vi "User.SettingsGui.vi"(11 "User in":i32(ring) caption="Operator" items=["-", "Admin", "Maciek"]) -> ()   [LabVIEW 2013]
uses:
  User.Global.vi
  User.SettingsGui.Action.ctl
  User.Level.ctl
  Tma.lib/array.llb/Select I32s from array.vi
  Tma.lib/array.llb/Select strings from array.vi
  EventLog/EventLog.New(array).vi
  Translator/Translator.Message.ctl
panel:
  out "_loop":i32(ring)=4
  in  "open?":bool
  in  "NewButton":bool
  in  "GuruPeriod":u32 caption="Guru Period Time [day]"
  in  "SetGuru":bool caption="Guru"
  in  "CancelButton":bool
  in  "UserLevel":T1 caption="User Level"
  in  "AutoLogOffTime":u32=1 caption="Auto Log-Off Time [min]" min=1 max=9999
  in  "RemoveButton":bool
  in  "ModifyButton":bool
  in  "AddButton":bool
  in  "UserName":string caption="Name"
  in  "pwd_Password2":string caption="Confirm Password"
  in  "pwd_Password":string caption="Password"
  in  "User":i32(ring) caption="Operator" items=["Service"=1, "Operator"=2]
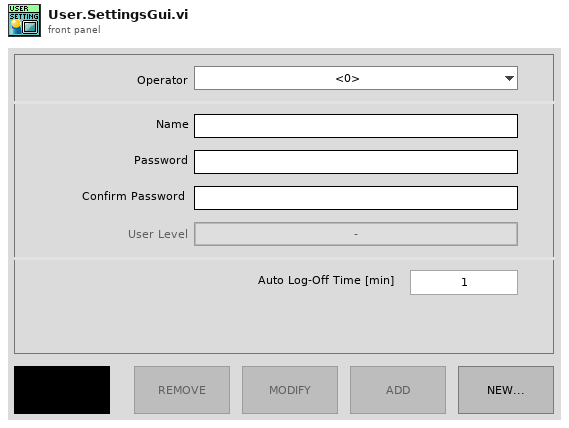
[diagram p1: front panel]
types:
  T1 = typedef "User.Level.ctl" = enum16{"-", "Operator", "Technician", "Administrator"}
  T2 = typedef "User.SettingsGui.Action.ctl" = enum32{"idle", "constructor", "destructor", "--- User Settings GUI ---", "check name & pass", "add user", "modify user", "remove user", "select user"}
  T3 = typedef "Translator.Message.ctl" = enum16{"-", "Event confirmed", "Log out", "Log in", "Shutdown", "Cancel", "Start", "Error %d >> %s", "Error %d >> %s >> %s", "Starting %s", "Quitting %s", "User %s level %s added", "User %s level %s deleted", "User %s level %s changed to %s", "Configured", "Initializing", "Quitting", "Loading", "Running", "Stopped", "Do you want to continue?", "Calibration", "Log out?", "System", "All", "IDLE", "Translating...%s", "Not found", "Alarm %s", "Restart is required to translate the application! Do you want to restart the PC?", "Restart cancelled. Be aware that some controls may not be fully translated until you restart the application.", "New version available!", "The software is up-to-date", "PC software will be updated after rebooting the PC. Do you want to reboot now?", "RT software will be updated. Make sure that no process is running. Do you want to reboot RT now?", "Updating RT firmware. Please wait...", "Update failed: %s", "Rebooting...", "Rebooting RT. Please wait...", "RT updated to version %s", "Timeout error during update. Check if RT is working", "Run", "Skip", "Abort", "Please wait...", "Database disconnected - changeover disabled!", "Put reference number...", "Folder '%s' is missing", "File '%s' is missing", "File '%s' is broken", "File '%s' is running", "Log file '%s' started", "Step '%s' added to log file", "Log file '%s' ended", "Test steps are missing", "Output %s = %.3f", "Process param '%s' not found in DB", "Process param '%s' wrong order", "Process param '%s' value %.3f out of limits (%.3f; %.3f)", "Step%d param '%s' not found in DB", "Step%d param '%s' wrong order", "Step%d param '%s' value %.3f out of limits (%.3f; %.3f)", "Step%d EV '%s' not found in DB", "Step%d EV '%s' wrong order", "Reference %d accepted", "Scan label failed", "Scan label failed. Error %d", "Scan label failed. Scanner disconnected", "Scan label: %s, %s", "Scan plate failed", "Scan plate failed. Wrong reference %d", "Scan plate failed. Serial number %d not unique", "Scan plate failed. Error %s", "Scan plate failed. Scanner disconnected", "Scan plate: %d", "DAQ.DO '%s' = %d", "DAQ.DI '%s' = %d->%d", "CPX.DO '%s' = %d", "CPX.DOvalve '%s' = %d", "CPX.DI '%s' = %d->%d", "Unable to move Door to %s position - timeout", "Unable to move Door to %s position - emergency button", "Unable to move Door to %s position - safety bar", "Unable to move Door to %s position - safety edge", "Unable to reset Emergency Circuit - emg button", "Unable to reset Emergency Circuit - safety bar", "Unable to set digital output '%s' = %d", "Unable to switch on Air Main Valve - timeout", "Unable to switch off Air Main Valve - timeout", "Unable to move Servo Lift to %s position - timeout", "Unable to move Servo Lift to %s position - air pressure off", "Unable to move Product Press to %s position - timeout", "Unable to move Product Press to %s position - air pressure off", "Unable to move Needles to %s position - timeout", "Unable to move Needles to %s position - air pressure off", "Unable to move Plugs to %s position - timeout", "Unable to move Plugs to %s position - air pressure off", "Unable to move Plugs to %s position - Plug Press not in Home position", "Unable to move Screw to %s position - timeout", "Unable to move Screw to %s position - air pressure off", "Unable to move Plug Revolver to %s position - timeout", "Unable to move Plug Revolver to %s position - air pressure off", "Unable to move Plug Revolver to %s position - Plug Press not in Home position", "Unable to reload Plug Revolver - magazine missing", "Unable to reload Plug Revolver - magazine empty", "Reloaded last plugs in Plug Revolver", "Unable to move Plug Press to %s position while getting plugs from revolver - timeout", "Unable to move Plug Press to %s position while pressing plugs into product - timeout", "Unable to move Plug Press to %s position - undefined position of Plugs", "Unable to move Plug Press to %s position - air pressure off", "Unable to move Stamp to %s position - timeout", "Unable to move Stamp to %s position - air pressure off", "Unable to move Vent Press to %s position - timeout", "Unable to move Vent Press to %s position - air pressure off", "Unable to move Terminal Press to %s position - timeout", "Unable to move Terminal Press to %s position - air pressure off"}
  T4 = enum32{"invalid app kind", "Development System", "Run Time System", "Student Edition", "Embedded LabVIEW", "Evaluation", "Custom"}
  T5 = enum8{"Enabled", "Disabled", "Disabled and Grayed Out"}
  T6 = typedef "User.Info.ctl" = cluster{"ID":i32, "Name":string, "Pass":string, "Level":T1, "Del":bool}
  T7 = typedef "LVStringsAndValuesArrayTypeDef_I32.ctl" = cluster{"String":string, "Value":i32}[]
  T8 = typedef "LVPositionTypeDef.ctl" = cluster{"Left":i32, "Top":i32}
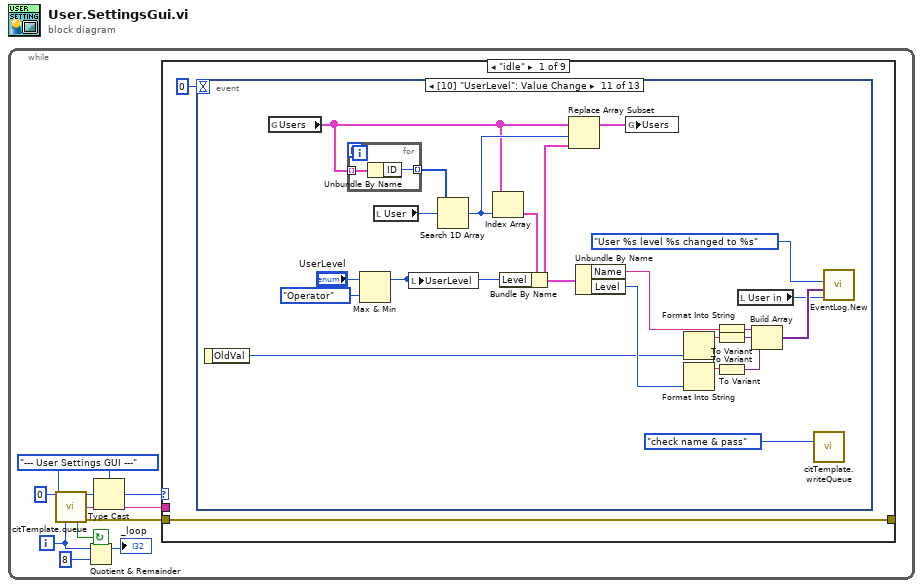
[diagram p0: block diagram]
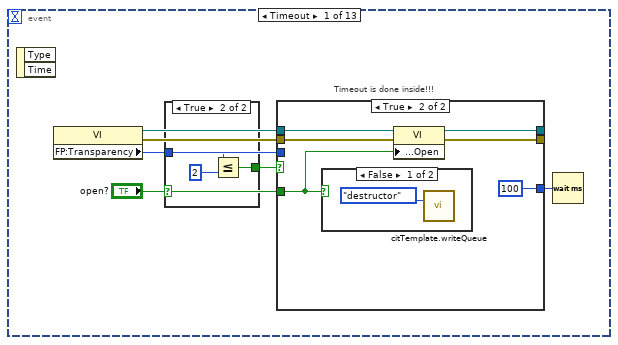
[diagram p2: hidden frame]
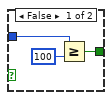
[diagram p3: hidden frame]
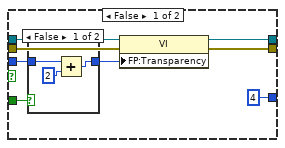
[diagram p4: hidden frame]
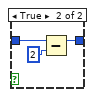
[diagram p5: hidden frame]
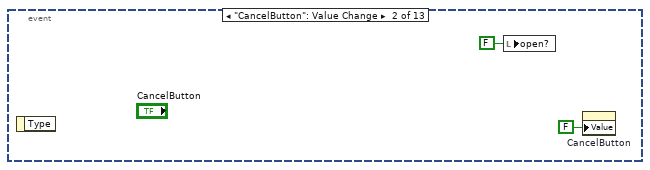
[diagram p7: hidden frame]
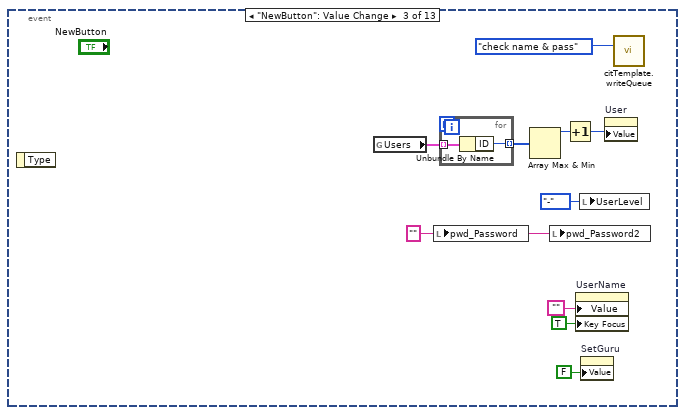
[diagram p8: hidden frame]
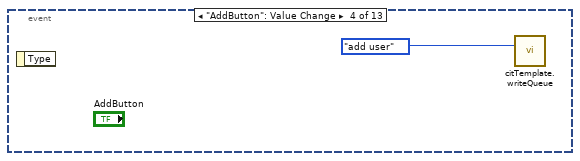
[diagram p9: hidden frame]
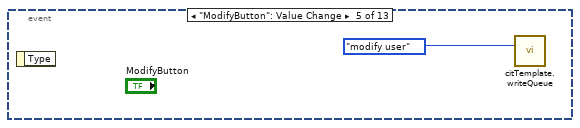
[diagram p10: hidden frame]
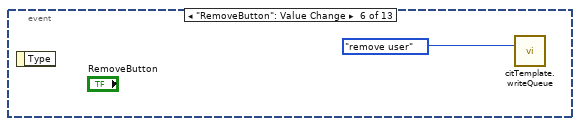
[diagram p11: hidden frame]
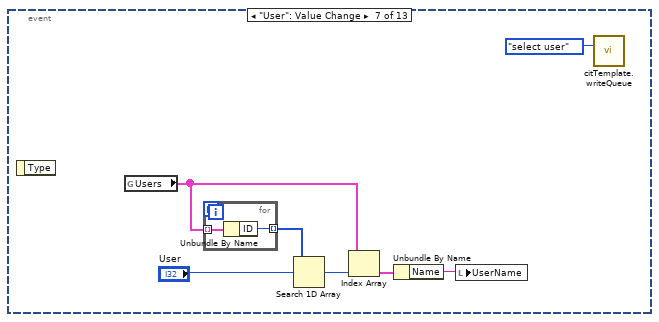
[diagram p12: hidden frame]
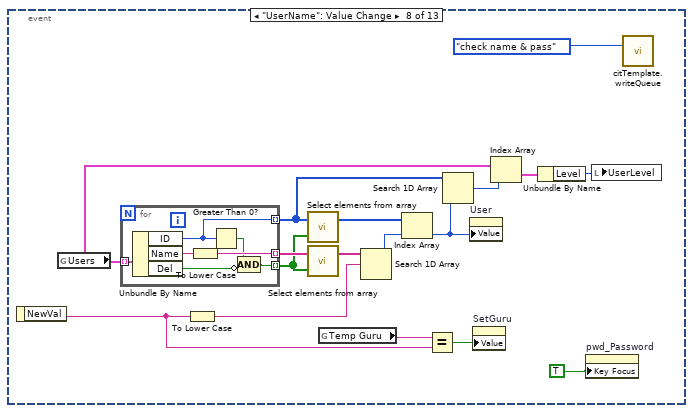
[diagram p13: hidden frame]
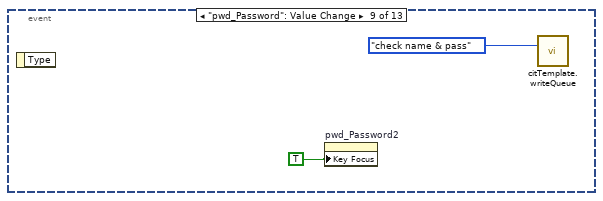
[diagram p14: hidden frame]
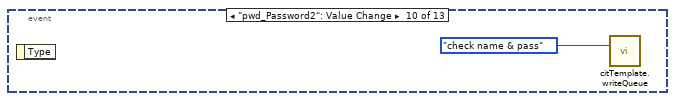
[diagram p15: hidden frame]
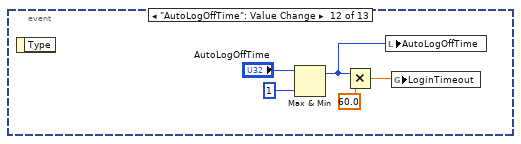
[diagram p16: hidden frame]
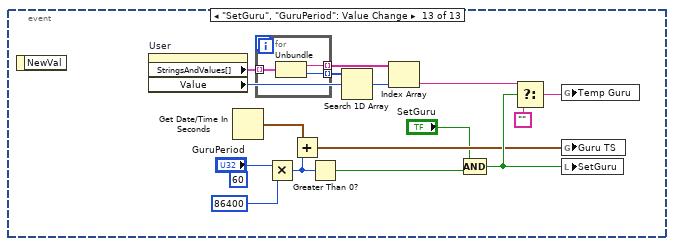
[diagram p17: hidden frame]
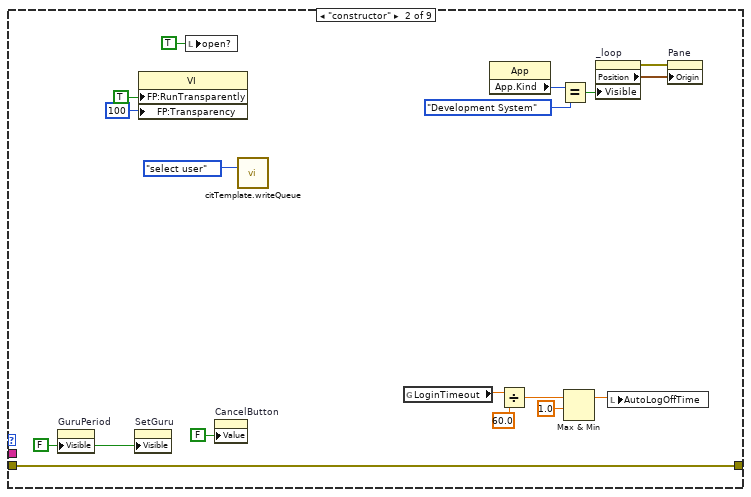
[diagram p18: hidden frame]
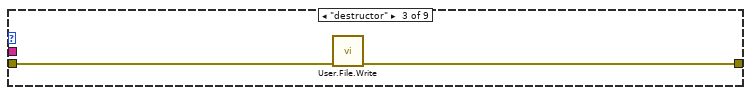
[diagram p19: hidden frame]
diagram:
  n1 = while {
    i -> [w1]
    stop <- w7 continue-if-true
    w6 = User.SettingsGui.Action."--- User Settings GUI ---" ("Action")
    n2 = call "citTemplate.queue.vi"("ms timeout (250 ms)"=0, "event enum"=w6, "iteration (-1)"=w1) -> ("event out"=w10:u32, "(flatten) data out"=w9:string, "continue"=w7:bool, "error out"=w8:errorcluster)  [unwired: 2 in, 7 out]
    n3 = Quotient & Remainder(x=w1, y=8) -> (x-y*floor(x/y)=→"_loop":i32)  [unwired: 1 out]
    n4 = Type Cast(type=w6, x=w10) -> (*(type *) &x=w5:T2)
    n5 = case shown="\"idle\"" w5 {
      tunnel: w9 -> [_ _ _ _ _ _ _ _ _]
      tunnel: w8 -> [w11 w147 w164 w166 w204 w259 w305 w332 w366]
      tunnel: [w11 w147 w165 w166 w204 w259 w305 w332 w366] -> _
      frame "idle" {
        n6 = event shown="[10] \"UserLevel\": Value Change" {
          selector: _ -> [_ _ _ _ _ _ _ _ _ _ _ _ _]
          dyn-events: _ -> [_ _ _ _ _ _ _ _ _ _ _ _ _]
          timeout: 0 -> [_ _ _ _ _ _ _ _ _ _ _ _ _]
          event Timeout {
            # "Timeout is done inside!!!"
            n7 = event-data() -> ()  [unwired: 1 in, 2 out]
            n8 = property class="VI"() -> (reference out=w16:refnum<vi>, error out=w15:errorcluster, "FP:Transparency"=w17:u8)  [unwired: 2 in]
            n9 = case shown="True" "open?" {
              tunnel: w17 -> [w20 w24]
              tunnel: [w19 w23] -> w18
              frame False {
                n10 = Greater Or Equal?(x=w20, y=u8 100) -> (x >= y?=w19:bool)
              }
              frame True {
                n11 = Less Or Equal?(x=w24, y=u8 2) -> (x <= y?=w23:bool)
              }
            }
            n12 = case shown="True" w18 {
              tunnel: w15 -> [w32 w44]
              tunnel: w16 -> [w31 w43]
              tunnel: w17 -> [w30 _]
              tunnel: "open?" -> [w29 w39]
              tunnel: [w27 w42] -> _
              tunnel: [w26 w41] -> _
              tunnel: [u32 4 ("milliseconds to wait") u32 100 ("ms timeout (250 ms)")] -> w13
              frame False {
                n13 = case shown="False" w29 {
                  tunnel: w30 -> [w35 w37]
                  tunnel: [w34 w36] -> w28
                  frame False {
                    n14 = Add(x=w35, y=u8 2 ("x")) -> (x+y=w34:u8)
                  }
                  frame True {
                    n15 = Subtract(x=w37, y=u8 2 ("x")) -> (x-y=w36:u8)
                  }
                }
                n16 = property class="VI"(reference=w31, error in=w32, "FP:Transparency"=w28) -> (reference out=w26:refnum<vi>, error out=w27:errorcluster)
              }
              frame True {
                n17 = case shown="False" w39 {
                  frame False {
                    n18 = call "citTemplate.writeQueue.vi"("event in (if not connected:all statemachine with data event)"=User.SettingsGui.Action."destructor" ("Action")) -> ()  [unwired: 4 in, 11 out]
                  }
                  frame True {
                  }
                }
                n19 = property class="VI"(reference=w43, error in=w44, "Front Panel.Open"=w39) -> (reference out=w41:refnum<vi>, error out=w42:errorcluster)
              }
            }
            n20 = Wait (ms)(milliseconds to wait=w13) -> ()  [unwired: 1 out]
          }
          event "CancelButton": Value Change {
            n21 = event-data() -> ()  [unwired: 1 in, 1 out]
            n22 = local write "open?"(FALSE ("open?")) -> ()
            n23 = property on="CancelButton" class="Bool (strict)"("Value"=FALSE ("CancelButton")) -> ()  [unwired: 2 in, 2 out]
          }
          event "NewButton": Value Change {
            w56 = "" ("Password")
            n24 = event-data() -> ()  [unwired: 1 in, 1 out]
            n25 = global read "User.Global.vi" "Users"() -> (w51:T6[])
            n26 = local write "pwd_Password"(w56) -> ()
            n27 = for {
              tunnel: w51 -> [w59] mode=indexing
              tunnel: [w58] -> w50 mode=indexing
              n28 = Unbundle By Name(w59) -> ("ID"=w58:i32)
            }
            n29 = Array Max & Min(array=w50) -> (max value=w49:i32)  [unwired: 3 out]
            n30 = local write "pwd_Password2"(w56) -> ()
            n31 = Increment(x=w49) -> (x+1=w48:i32)
            n32 = property on="UserName" class="Str"("Value"="", "Key Focus"=TRUE) -> ()  [unwired: 2 in, 2 out]
            n33 = local write "UserLevel"(User.Level."-" ("UserLevel")) -> ()
            n34 = property on="SetGuru" class="Bool (strict)"("Value"=FALSE ("SetGuru")) -> ()  [unwired: 2 in, 2 out]
            n35 = property on="User" class="Ring (strict)"("Value"=w48) -> ()  [unwired: 2 in, 2 out]
            n36 = call "citTemplate.writeQueue.vi"("event in (if not connected:all statemachine with data event)"=User.SettingsGui.Action."check name & pass" ("Action")) -> ()  [unwired: 14 in, 1 out]
          }
          event "AddButton": Value Change {
            n37 = event-data() -> ()  [unwired: 1 in, 1 out]
            n38 = call "citTemplate.writeQueue.vi"("event in (if not connected:all statemachine with data event)"=User.SettingsGui.Action."add user" ("Action")) -> ()  [unwired: 14 in, 1 out]
          }
          event "ModifyButton": Value Change {
            n39 = event-data() -> ()  [unwired: 1 in, 1 out]
            n40 = call "citTemplate.writeQueue.vi"("event in (if not connected:all statemachine with data event)"=User.SettingsGui.Action."modify user" ("Action")) -> ()  [unwired: 14 in, 1 out]
          }
          event "RemoveButton": Value Change {
            n41 = event-data() -> ()  [unwired: 1 in, 1 out]
            n42 = call "citTemplate.writeQueue.vi"("event in (if not connected:all statemachine with data event)"=User.SettingsGui.Action."remove user" ("Action")) -> ()  [unwired: 14 in, 1 out]
          }
          event "User": Value Change {
            n43 = event-data() -> ()  [unwired: 1 in, 1 out]
            n44 = global read "User.Global.vi" "Users"() -> (w65:T6[])
            n45 = for {
              tunnel: w65 -> [w71] mode=indexing
              tunnel: [w70] -> w67 mode=indexing
              n46 = Unbundle By Name(w71) -> ("ID"=w70:i32)
            }
            n47 = Search 1D Array(1D array=w67, element="User") -> (index of element=w66:i32)  [unwired: 1 in]
            n48 = Index Array(array=w65, index=w66) -> (element=w64:T6)
            n49 = Unbundle By Name(w64) -> ("Name"=w68:string)
            n50 = local write "UserName"(w68) -> ()
            n51 = call "citTemplate.writeQueue.vi"("event in (if not connected:all statemachine with data event)"=User.SettingsGui.Action."select user" ("Action")) -> ()  [unwired: 14 in, 1 out]
          }
          event "UserName": Value Change {
            n52 = event-data() -> ("NewVal"=w77:string)  [unwired: 1 in]
            n53 = global read "User.Global.vi" "Users"() -> (w73:T6[])
            n54 = for {
              tunnel: w73 -> [w95] mode=indexing
              tunnel: [w93] -> w84 mode=indexing
              tunnel: [w91] -> w72 mode=indexing
              tunnel: [w89] -> w75 mode=indexing
              n55 = Unbundle By Name(w95) -> ("ID"=w89:i32, "Name"=w94:string, "Del"=w92:bool)
              n56 = To Lower Case(string=w94) -> (all lower case string=w93:string)
              n57 = Greater Than 0?(x=w89) -> (x > 0?=w90:bool)
              n58 = Compound Arithmetic op=AND(w90, invert w92) -> (w91:bool)
            }
            n59 = To Lower Case(string=w77) -> (all lower case string=w87:string)
            n60 = call-poly "Select elements from array.vi"("selection array"=w72, "I32s"=w75) -> ("selected I32s"=w82:i32[])  [unwired: 1 in]
            n61 = call-poly "Select elements from array.vi"("selection array"=w72, "strings"=w84) -> ("selected strings"=w83:string[])  [unwired: 1 in]
            n62 = global read "User.Global.vi" "Temp Guru"() -> (w80:string)
            n63 = Search 1D Array(1D array=w83, element=w87) -> (index of element=w81:i32)  [unwired: 1 in]
            n64 = Index Array(array=w82, index=w81) -> (element=w76:i32)
            n65 = Equal?(x=w80, y=w77) -> (x = y?=w79:bool)
            n66 = Search 1D Array(1D array=w75, element=w76) -> (index of element=w74:i32)  [unwired: 1 in]
            n67 = property on="User" class="Ring (strict)"("Value"=w76) -> ()  [unwired: 2 in, 2 out]
            n68 = property on="SetGuru" class="Bool (strict)"("Value"=w79) -> ()  [unwired: 2 in, 2 out]
            n69 = Index Array(array=w73, index=w74) -> (element=w86:T6)
            n70 = Unbundle By Name(w86) -> ("Level"=w85:T1)
            n71 = property on="pwd_Password" class="Str"("Key Focus"=TRUE) -> ()  [unwired: 2 in, 2 out]
            n72 = local write "UserLevel"(w85) -> ()
            n73 = call "citTemplate.writeQueue.vi"("event in (if not connected:all statemachine with data event)"=User.SettingsGui.Action."check name & pass" ("Action")) -> ()  [unwired: 14 in, 1 out]
          }
          event "pwd_Password": Value Change {
            n74 = event-data() -> ()  [unwired: 1 in, 1 out]
            n75 = property on="pwd_Password2" class="Str"("Key Focus"=TRUE) -> ()  [unwired: 2 in, 2 out]
            n76 = call "citTemplate.writeQueue.vi"("event in (if not connected:all statemachine with data event)"=User.SettingsGui.Action."check name & pass" ("Action")) -> ()  [unwired: 14 in, 1 out]
          }
          event "pwd_Password2": Value Change {
            n77 = event-data() -> ()  [unwired: 1 in, 1 out]
            n78 = call "citTemplate.writeQueue.vi"("event in (if not connected:all statemachine with data event)"=User.SettingsGui.Action."check name & pass" ("Action")) -> ()  [unwired: 14 in, 1 out]
          }
          event Value Change {
            n79 = event-data() -> ("OldVal"=w101:T1)  [unwired: 1 in]
            n80 = global read "User.Global.vi" "Users"() -> (w112:T6[])
            n81 = for {
              tunnel: w112 -> [w122] mode=indexing
              tunnel: [w121] -> w115 mode=indexing
              n82 = Unbundle By Name(w122) -> ("ID"=w121:i32)
            }
            n83 = Max & Min(x="UserLevel", y=User.Level."Operator") -> (max(x,y)=w118:u16)  [unwired: 1 out]
            n84 = local read "User"() -> (w114:i32)
            n85 = local write "UserLevel"(w118) -> ()
            n86 = Search 1D Array(1D array=w115, element=w114) -> (index of element=w113:i32)  [unwired: 1 in]
            n87 = Index Array(array=w112, index=w113) -> (element=w104:T6)
            n88 = Bundle By Name(cluster=w104, "Level"=w118) -> (w103:T6)
            n89 = Replace Array Subset(array=w112, new element=w103, index=w113) -> (w116:T6[])
            n90 = Unbundle By Name(w103) -> ("Name"=w105:string, "Level"=w102:T1)
            n91 = global write "User.Global.vi" "Users"(w116) -> ()
            n92 = Format Into String(w101) -> (resulting string=w110:string)  [unwired: 3 in, 1 out]
            n93 = Format Into String(w102) -> (resulting string=w100:string)  [unwired: 3 in, 1 out]
            n94 = To Variant(anything=w105) -> (Variant=w109:variant)
            n95 = To Variant(anything=w110) -> (Variant=w108:variant)
            n96 = To Variant(anything=w100) -> (Variant=w99:variant)
            n97 = local read "User in"() -> (w106:i32)
            n98 = Build Array(w109, w108, w99) -> (w107:variant[])
            n99 = call "citTemplate.writeQueue.vi"("event in (if not connected:all statemachine with data event)"=User.SettingsGui.Action."check name & pass" ("Action")) -> ()  [unwired: 14 in, 1 out]
            n100 = call-poly "EventLog.New.vi"("error in (no error)"=w106, "Arguments"=w107, "Message (-)"=Translator.Message."User %s level %s changed to %s") -> ()  [unwired: 7 in, 2 out]
          }
          event "AutoLogOffTime": Value Change {
            n101 = event-data() -> ()  [unwired: 1 in, 1 out]
            n102 = Max & Min(x="AutoLogOffTime", y=u32 1 ("lower limit")) -> (max(x,y)=w127:u32)  [unwired: 1 out]
            n103 = Multiply(x=w127, y=60.0 ("x")) -> (x*y=w123:dbl)
            n104 = local write "AutoLogOffTime"(w127) -> ()
            n105 = global write "User.Global.vi" "LoginTimeout"(w123) -> ()
          }
          event "SetGuru", "GuruPeriod": Value Change {
            (unwired) u32 60 ("y")
            n106 = event-data() -> ()  [unwired: 1 in, 1 out]
            n107 = property on="User" class="Ring (strict)"() -> ("StringsAndValues[]"=w133:T7, "Value"=w131:i32)  [unwired: 2 in, 2 out]
            n108 = Get Date/Time In Seconds() -> (seconds since 1Jan1904=w134:timestamp)
            n109 = for {
              tunnel: w133 -> [w146] mode=indexing
              tunnel: [w145] -> w132 mode=indexing
              tunnel: [w144] -> w130 mode=indexing
              n110 = Unbundle(w146) -> ("String"=w144:string, "Value"=w145:i32)
            }
            n111 = Multiply(x="GuruPeriod", y=u32 86400) -> (x*y=w135:u32)
            n112 = Add(x=w134, y=w135) -> (x+y=w140:timestamp)
            n113 = Greater Than 0?(x=w135) -> (x > 0?=w137:bool)
            n114 = Search 1D Array(1D array=w132, element=w131) -> (index of element=w129:i32)  [unwired: 1 in]
            n115 = Index Array(array=w130, index=w129) -> (element=w128:string)
            n116 = Compound Arithmetic op=AND("SetGuru", w137) -> (w141:bool)
            n117 = Select(t=w128, s=w141, f="") -> (s? t:f=w136:string)
            n118 = global write "User.Global.vi" "Temp Guru"(w136) -> ()
            n119 = global write "User.Global.vi" "Guru TS"(w140) -> ()
            n120 = local write "SetGuru"(w141) -> ()
          }
        }
      }
      frame "constructor" {
        w157 = FALSE ("Visible")
        n121 = property on="GuruPeriod" class="DigNum (strict)"("Visible"=w157) -> ()  [unwired: 2 in, 2 out]
        n122 = property on="SetGuru" class="Bool (strict)"("Visible"=w157) -> ()  [unwired: 2 in, 2 out]
        n123 = property class="VI"("FP:RunTransparently"=TRUE ("Front Panel Window:Run VI Transparently"), "FP:Transparency"=u8 100 ("Front Panel Window:Transparency")) -> ()  [unwired: 2 in, 2 out]
        n124 = local write "open?"(TRUE ("open?")) -> ()
        n125 = property on="CancelButton" class="Bool (strict)"("Value"=FALSE ("CancelButton")) -> ()  [unwired: 2 in, 2 out]
        n126 = call "citTemplate.writeQueue.vi"("event in (if not connected:all statemachine with data event)"=User.SettingsGui.Action."select user" ("Action")) -> ()  [unwired: 14 in, 1 out]
        n127 = global read "User.Global.vi" "LoginTimeout"() -> (w156:dbl)
        n128 = property class="App"() -> ("App.Kind"=w150:T4)  [unwired: 2 in, 2 out]
        n129 = Divide(x=w156, y=60.0 ("x")) -> (x/y=w160:dbl)
        n130 = Equal?(x=w150, y=T4."Development System") -> (x = y?=w148:bool)
        n131 = Max & Min(x=w160, y=1.0 ("lower limit")) -> (max(x,y)=w163:dbl)  [unwired: 1 out]
        n132 = property on="_loop" class="Ring (strict)"("Visible"=w148) -> (error out=w152:errorcluster, "Position"=w151:T8)  [unwired: 2 in, 1 out]
        n133 = local write "AutoLogOffTime"(w163) -> ()
        n134 = property on="Pane" class="Pane"(error in=w152, "Origin"=w151) -> ()  [unwired: 1 in, 2 out]
      }
      frame "destructor" {
        n135 = call "User.File.Write.vi"("error in (no error)"=w164) -> ("error out"=w165:errorcluster)  [unwired: 10 in]
      }
      frame "--- User Settings GUI ---" {
      }
      frame "check name & pass" {
        w194 = User.Level."Administrator" ("x")
        w225 = T5."Disabled and Grayed Out" ("Disabled")
        n136 = global read "User.Global.vi" "Users"() -> (w218:T6[])
        n137 = global read "User.Global.vi" "DefaultUser"() -> (w175:string)
        n138 = global read "User.Global.vi" "Admin User"() -> (w173:string)
        n139 = local read "UserLevel"() -> (w192:T1)
        n140 = for {
          tunnel: w218 -> [w245] mode=indexing
          tunnel: [w243] -> w174 mode=indexing
          tunnel: [w242] -> w212 mode=indexing
          tunnel: [w238] -> w169 mode=indexing
          tunnel: w194 -> [w240]
          tunnel: [w237] -> w193 mode=indexing
          i -> [w236]
          n141 = Greater Than 0?(x=w236) -> (x > 0?=w235:bool)
          n142 = Unbundle By Name(w245) -> ("Level"=w241:T1, "Del"=w238:bool, "Name"=w244:string, "Pass"=w242:string)
          n143 = Equal?(x=w240, y=w241) -> (x = y?=w239:bool)
          n144 = To Lower Case(string=w244) -> (all lower case string=w243:string)
          n145 = Compound Arithmetic op=AND(w235, w239, invert w238) -> (w237:bool)
        }
        n146 = To Lower Case(string="UserName") -> (all lower case string=w213:string)
        n147 = call "MD5 string.vi"("Message String"="pwd_Password") -> ("MD5 message-digest"=w210:string)  [unwired: 10 in]
        n148 = Not Equal?(x="pwd_Password", y="pwd_Password2") -> (x != y?=w229:bool)
        n149 = Empty String/Path?(string/path="pwd_Password") -> (empty?=w228:bool)
        n150 = Equal To 0?(x="User in") -> (x = 0?=w171:bool)
        n151 = Boolean To (0,1)(Boolean=w193) -> (0, 1=w199:i16[])
        n152 = Search 1D Array(1D array=w212, element=w210) -> (index of element=w209:i32)  [unwired: 1 in]
        n153 = Delete From Array(array=w169, index=0) -> (array with subset deleted=w168:bool[])  [unwired: 1 in, 1 out]
        n154 = To Lower Case(string=w175) -> (all lower case string=w177:string)
        n155 = To Lower Case(string=w173) -> (all lower case string=w176:string)
        n156 = Search 1D Array(1D array=w174, element=w213) -> (index of element=w170:i32)  [unwired: 1 in]
        n157 = Array Size(array=w174) -> (size(s)=w224:i32)
        n158 = To Long Integer(number=w199) -> (32bit integer=w198:i32[])
        n159 = Not Equal?(x=w170, y=w209) -> (x != y?=w208:bool)
        n160 = Index Array(array=w169, index=w170) -> (element=w205:bool)
        n161 = Greater Or Equal To 0?(x=w209) -> (x >= 0?=w207:bool)
        n162 = Equal?(x=w213, y=w177) -> (x = y?=w186:bool)
        n163 = Equal?(x=w213, y=w176) -> (x = y?=w179:bool)
        n164 = Add Array Elements(numeric array=w198) -> (sum=w197:i32)
        n165 = Less Or Equal To 0?(x=w224) -> (x <= 0?=w183:bool)
        n166 = Greater Or Equal To 0?(x=w170) -> (x >= 0?=w215:bool)
        n167 = Less Or Equal To 0?(x=w192) -> (x <= 0?=w203:bool)
        n168 = Compound Arithmetic op=AND(w208, w207) -> (w206:bool)
        n169 = And Array Elements(Boolean array=w168) -> (logical AND=w184:bool)
        n170 = Equal?(x=1, y=w197) -> (x = y?=w195:bool)
        n171 = Equal?(x=w194, y=w192) -> (x = y?=w185:bool)
        n172 = Compound Arithmetic op=AND(invert w205, w215) -> (w178:bool)
        n173 = Compound Arithmetic op=OR(w184, w183) -> (w182:bool)
        n174 = Compound Arithmetic op=AND(w185, w195) -> (w180:bool)
        n175 = Compound Arithmetic op=OR(w182, w186, w179, w228, w229, w206) -> (w227:bool)
        n176 = Compound Arithmetic op=OR(w178, w186, w179, w228, w229, w203) -> (w232:bool)
        n177 = Compound Arithmetic op=OR(w180, w182) -> (w181:bool)
        n178 = Compound Arithmetic op=AND(w178, invert w227, invert w203) -> (w226:bool)
        n179 = property on="SetGuru" class="Bool (strict)"() -> ("Value"=w187:bool)  [unwired: 2 in, 2 out]
        n180 = Compound Arithmetic op=AND(w171, w185, invert w182, w178) -> (w191:bool)
        n181 = Select(t=w225, s=w232, f=T5."Enabled" ("Disabled")) -> (s? t:f=w234:T5)
        n182 = Select(t=T5."Disabled and Grayed Out" ("Disabled"), s=w181, f=T5."Enabled" ("Disabled")) -> (s? t:f=w222:T5)
        n183 = property on="GuruPeriod" class="DigNum (strict)"("Visible"=w191) -> ()  [unwired: 2 in, 2 out]
        n184 = Select(t=T5."Enabled" ("Disabled"), s=w226, f=w225) -> (s? t:f=w231:T5)
        n185 = Select(t=T5."Disabled and Grayed Out" ("Disabled"), s=w182, f=T5."Enabled" ("Disabled")) -> (s? t:f=w221:T5)
        n186 = Compound Arithmetic op=AND(invert w185, w187) -> (w190:bool)
        n187 = Select(t=T5."Disabled and Grayed Out" ("Disabled"), s=w180, f=T5."Enabled" ("Disabled")) -> (s? t:f=w202:T5)
        n188 = property on="User" class="Ring (strict)"("DisabledEnum"=w221) -> ()  [unwired: 2 in, 2 out]
        n189 = property on="ModifyButton" class="Bool"("DisabledEnum"=w231) -> ()  [unwired: 2 in, 2 out]
        n190 = property on="AddButton" class="Bool"("DisabledEnum"=w234) -> ()  [unwired: 2 in, 2 out]
        n191 = property on="RemoveButton" class="Bool"("DisabledEnum"=w222) -> ()  [unwired: 2 in, 2 out]
        n192 = Select(t=FALSE, s=w190, f=w187) -> (s? t:f=w188:bool)
        n193 = property on="UserLevel" class="Enum (strict)"("DisabledEnum"=w202) -> ()  [unwired: 2 in, 2 out]
        n194 = property on="SetGuru" class="Bool (strict)"("Value"=w188, "Visible"=w191) -> ()  [unwired: 2 in, 2 out]
      }
      frame "add user" {
        n195 = global read "User.Global.vi" "Users"() -> (w262:T6[])
        n196 = for {
          tunnel: w262 -> [w288] mode=indexing
          tunnel: [w286] -> w264 mode=indexing
          tunnel: [w285] -> w258 mode=indexing
          n197 = Unbundle By Name(w288) -> ("Name"=w287:string, "ID"=w285:i32)
          n198 = To Lower Case(string=w287) -> (all lower case string=w286:string)
        }
        n199 = local read "pwd_Password"() -> (w266:string)
        n200 = local read "UserName"() -> (w250:string)
        n201 = local read "UserLevel"() -> (w252:T1)
        n202 = Array Max & Min(array=w258) -> (max value=w257:i32)  [unwired: 3 out]
        n203 = call "MD5 string.vi"("Message String"=w266) -> ("MD5 message-digest"=w255:string)  [unwired: 10 in]
        n204 = To Lower Case(string=w250) -> (all lower case string=w260:string)
        n205 = Increment(x=w257) -> (x+1=w256:i32)
        n206 = Search 1D Array(1D array=w264, element=w260) -> (index of element=w263:i32)  [unwired: 1 in]
        n207 = case shown="Default" w263 {
          selector: w263 -> [w272 w282]
          tunnel: [w274 w284] -> w261
          tunnel: w262 -> [w273 w281]
          tunnel: w256 -> [_ w283]
          tunnel: w250 -> [_ w275]
          tunnel: w255 -> [w269 w276]
          tunnel: w252 -> [w268 w277]
          tunnel: FALSE ("Del") -> [w267 w278]
          frame 0.. {
            # "modify user"
            n208 = Index Array(array=w273, index=w272) -> (element=w271:T6)
            n209 = Bundle By Name(cluster=w271, "Pass"=w269, "Level"=w268, "Del"=w267) -> (w270:T6)
            n210 = Replace Array Subset(array=w273, new element=w270, index=w272) -> (w274:T6[])
          }
          frame Default {
            # "add user"
            n211 = Index Array(array=w281, index=w282) -> (element=w280:T6)
            n212 = Bundle By Name(cluster=w280, "ID"=w283, "Name"=w275, "Pass"=w276, "Level"=w277, "Del"=w278) -> (w279:T6)
            n213 = Build Array (concatenate)(w281, w279) -> (w284:T6[])
          }
        }
        n214 = Format Into String(w252) -> (resulting string=w251:string)  [unwired: 3 in, 1 out]
        n215 = To Variant(anything=w250) -> (Variant=w249:variant)
        n216 = To Variant(anything=w251) -> (Variant=w248:variant)
        n217 = global write "User.Global.vi" "Users"(w261) -> ()
        n218 = local read "User in"() -> (w246:i32)
        n219 = Build Array(w249, w248) -> (w247:variant[])
        n220 = call "citTemplate.writeQueue.vi"("event in (if not connected:all statemachine with data event)"=User.SettingsGui.Action."select user" ("Action")) -> ()  [unwired: 14 in, 1 out]
        n221 = call-poly "EventLog.New.vi"("error in (no error)"=w246, "Arguments"=w247, "Message (-)"=Translator.Message."User %s level %s added") -> ()  [unwired: 7 in, 2 out]
      }
      frame "modify user" {
        n222 = global read "User.Global.vi" "Users"() -> (w299:T6[])
        n223 = local read "pwd_Password"() -> (w308:string)
        n224 = for {
          tunnel: w299 -> [w310] mode=indexing
          tunnel: [w309] -> w302 mode=indexing
          n225 = Unbundle By Name(w310) -> ("ID"=w309:i32)
        }
        n226 = local read "UserLevel"() -> (w292:T1)
        n227 = local read "User"() -> (w301:i32)
        n228 = call "MD5 string.vi"("Message String"=w308) -> ("MD5 message-digest"=w307:string)  [unwired: 10 in]
        n229 = Search 1D Array(1D array=w302, element=w301) -> (index of element=w300:i32)  [unwired: 1 in]
        n230 = Index Array(array=w299, index=w300) -> (element=w291:T6)
        n231 = Bundle By Name(cluster=w291, "Pass"=w307, "Level"=w292) -> (w289:T6)
        n232 = Unbundle By Name(w289) -> ("Name"=w290:string)
        n233 = Replace Array Subset(array=w299, new element=w289, index=w300) -> (w303:T6[])
        n234 = global write "User.Global.vi" "Users"(w303) -> ()
        n235 = Format Into String(w292) -> (resulting string=w297:string)  [unwired: 3 in, 1 out]
        n236 = To Variant(anything=w290) -> (Variant=w296:variant)
        n237 = To Variant(anything=w297) -> (Variant=w295:variant)
        n238 = local read "User in"() -> (w293:i32)
        n239 = Build Array(w296, w295) -> (w294:variant[])
        n240 = call-poly "EventLog.New.vi"("error in (no error)"=w293, "Arguments"=w294, "Message (-)"=Translator.Message."User %s level %s changed to %s") -> ()  [unwired: 7 in, 2 out]
        n241 = call "citTemplate.writeQueue.vi"("event in (if not connected:all statemachine with data event)"=User.SettingsGui.Action."select user" ("Action")) -> ()  [unwired: 14 in, 1 out]
        n242 = call "citTemplate.writeQueue.vi"("event in (if not connected:all statemachine with data event)"=User.SettingsGui.Action."select user" ("Action")) -> ()  [unwired: 14 in, 1 out]
      }
      frame "remove user" {
        w336 = "" ("Password")
        n243 = global read "User.Global.vi" "Users"() -> (w328:T6[])
        n244 = for {
          tunnel: w328 -> [w339] mode=indexing
          tunnel: [w338] -> w331 mode=indexing
          n245 = Unbundle By Name(w339) -> ("ID"=w338:i32)
        }
        n246 = local read "User"() -> (w330:i32)
        n247 = local write "pwd_Password"(w336) -> ()
        n248 = Search 1D Array(1D array=w331, element=w330) -> (index of element=w329:i32)  [unwired: 1 in]
        n249 = local write "pwd_Password2"(w336) -> ()
        n250 = Index Array(array=w328, index=w329) -> (element=w313:T6)
        n251 = Bundle By Name(cluster=w313, "Del"=TRUE) -> (w334:T6)
        n252 = global read "User.Global.vi" "Temp Guru"() -> (w326:string)
        n253 = global read "User.Global.vi" "Guru TS"() -> (w320:timestamp)
        n254 = Unbundle By Name(w313) -> ("Name"=w327:string)
        n255 = Replace Array Subset(array=w328, new element=w334, index=w329) -> (w333:T6[])
        n256 = Unbundle By Name(w313) -> ("Name"=w312:string, "Level"=w311:T1)
        n257 = Not Equal?(x=w326, y=w327) -> (x != y?=w324:bool)
        n258 = global write "User.Global.vi" "Users"(w333) -> ()
        n259 = Select(t=w320, s=w324, f=timestamp(0 s since 1904-01-01)) -> (s? t:f=w321:timestamp)
        n260 = Select(t=w326, s=w324, f="") -> (s? t:f=w325:string)
        n261 = Format Into String(w311) -> (resulting string=w318:string)  [unwired: 3 in, 1 out]
        n262 = global write "User.Global.vi" "Temp Guru"(w325) -> ()
        n263 = global write "User.Global.vi" "Guru TS"(w321) -> ()
        n264 = To Variant(anything=w312) -> (Variant=w317:variant)
        n265 = To Variant(anything=w318) -> (Variant=w316:variant)
        n266 = local read "User in"() -> (w314:i32)
        n267 = Build Array(w317, w316) -> (w315:variant[])
        n268 = call-poly "EventLog.New.vi"("error in (no error)"=w314, "Arguments"=w315, "Message (-)"=Translator.Message."User %s level %s deleted") -> ()  [unwired: 7 in, 2 out]
        n269 = call "citTemplate.writeQueue.vi"("event in (if not connected:all statemachine with data event)"=User.SettingsGui.Action."select user" ("Action")) -> ()  [unwired: 14 in, 1 out]
      }
      frame "select user" {
        w352 = "" ("Password")
        n270 = global read "User.Global.vi" "Users"() -> (w346:T6[])
        n271 = global read "User.Global.vi" "Guru TS"() -> (w360:timestamp)
        n272 = for {
          tunnel: w346 -> [w387] mode=indexing
          tunnel: [w383] -> w371 mode=indexing
          tunnel: [w384] -> w372 mode=indexing
          tunnel: [w382] -> w345 mode=indexing
          n273 = Unbundle By Name(w387) -> ("ID"=w382:i32, "Name"=w383:string, "Del"=w386:bool)
          n274 = Greater Than 0?(x=w382) -> (x > 0?=w385:bool)
          n275 = Compound Arithmetic op=AND(w385, invert w386) -> (w384:bool)
        }
        n276 = Get Date/Time In Seconds() -> (seconds since 1Jan1904=w359:timestamp)
        n277 = Subtract(x=w360, y=w359) -> (x-y=w357:dbl)
        n278 = Greater?(x=w360, y=w359) -> (0:w363:bool)
        n279 = global read "User.Global.vi" "Temp Guru"() -> (w362:string)
        n280 = Divide(x=w357, y=86400.0) -> (x/y=w355:dbl)
        n281 = local read "UserName"() -> (w367:string)
        n282 = Max & Min(x=w355, y=0.0) -> (max(x,y)=w354:dbl)  [unwired: 1 out]
        n283 = Round Toward +Infinity(x=w354) -> (ceil(x): smallest int >= x=w356:dbl)
        n284 = Select(t=w362, s=w363, f="") -> (s? t:f=w351:string)
        n285 = Select(t=w360, s=w363, f=timestamp(0 s since 1904-01-01)) -> (s? t:f=w358:timestamp)
        n286 = call-poly "Select elements from array.vi"("selection array"=w372, "strings"=w371) -> ("selected strings"=w342:string[])  [unwired: 1 in]
        n287 = call-poly "Select elements from array.vi"("selection array"=w372, "I32s"=w345) -> ("selected I32s"=w349:i32[])  [unwired: 1 in]
        n288 = Search 1D Array(1D array=w342, element=w367) -> (index of element=w348:i32)  [unwired: 1 in]
        n289 = property on="GuruPeriod" class="DigNum (strict)"("Value"=w356) -> ()  [unwired: 2 in, 2 out]
        n290 = global write "User.Global.vi" "Temp Guru"(w351) -> ()
        n291 = global write "User.Global.vi" "Guru TS"(w358) -> ()
        n292 = for {
          tunnel: w342 -> [w381] mode=indexing
          tunnel: w349 -> [w380] mode=indexing
          tunnel: [w379] -> w369 mode=indexing
          n293 = Bundle("Ping"=w381, "Ping"=w380) -> (w379:cluster{"Ping":string, "Ping":i32})  [unwired: 1 in]
        }
        n294 = Index Array(array=w349, index=w348) -> (element=w347:i32)
        n295 = Max & Min(x=w347, y=1) -> (max(x,y)=w341:i32)  [unwired: 1 out]
        n296 = Array Size(array=w369) -> (size(s)=w378:i32)
        n297 = Less Or Equal To 0?(x=w378) -> (x <= 0?=w377:bool)
        n298 = Select(t=T5."Disabled and Grayed Out" ("Disabled"), s=w377, f=T5."Enabled" ("Disabled")) -> (s? t:f=w375:T5)
        n299 = local write "pwd_Password"(w352) -> ()
        n300 = Search 1D Array(1D array=w345, element=w341) -> (index of element=w344:i32)  [unwired: 1 in]
        n301 = Index Array(array=w346, index=w344) -> (element=w343:T6)
        n302 = property on="User" class="Ring (strict)"("StringsAndValues[]"=w369, "DisabledEnum"=w375, "Value"=w341) -> ()  [unwired: 2 in, 2 out]
        n303 = Unbundle By Name(w343) -> ("Name"=w340:string, "Level"=w373:T1)
        n304 = local write "pwd_Password2"(w352) -> ()
        n305 = local write "UserName"(w340) -> ()
        n306 = local write "UserLevel"(w373) -> ()
        n307 = call "citTemplate.writeQueue.vi"("event in (if not connected:all statemachine with data event)"=User.SettingsGui.Action."check name & pass" ("Action")) -> ()  [unwired: 14 in, 1 out]
        n308 = call "citTemplate.writeQueue.vi"("event in (if not connected:all statemachine with data event)"=User.SettingsGui.Action."check name & pass" ("Action")) -> ()  [unwired: 14 in, 1 out]
      }
    }
  }
